vi "LocateDevices.vi"() -> ()   [LabVIEW 2017]
uses:
  D:/upwork/Laser Measurement Tool/Topas4PublicAPI/NET_SDK/Topas4Lib.dll
  Topas4PublicAPI/NET_SDK/Topas4Lib.dll
panel:
  out "Found devices info:":T1(array[cluster])
  out "OPA devices found:":i32
  # "Find OPA device test"
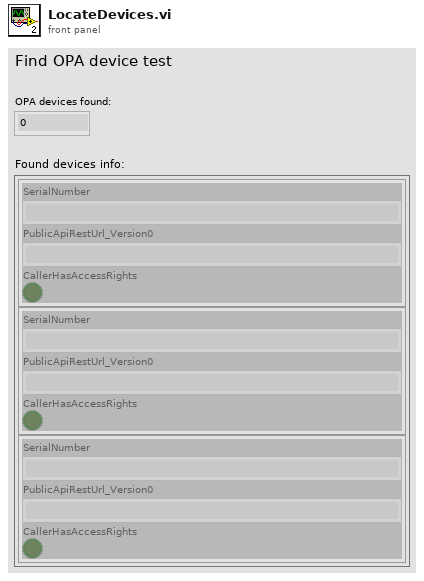
[diagram p1: front panel]
types:
  T1 = cluster{"SerialNumber":string, "PublicApiRestUrl_Version0":string, "CallerHasAccessRights":bool}[]
  T2 = cluster{"SerialNumber":string, "PublicApiRestUrl_Version0":string, "CallerHasAccessRights":bool}
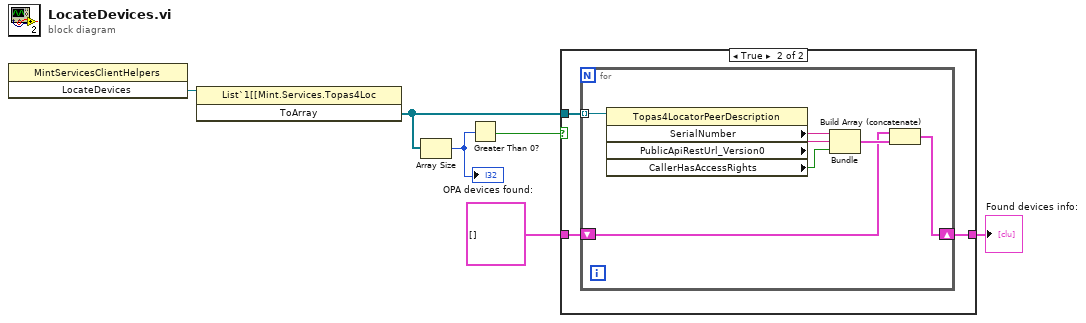
[diagram p0: block diagram]
diagram:
  n1 = invoke class="MintServicesClientHelpers" method="LocateDevices"() -> ("LocateDevices"=w6:refnum<k24>)  [unwired: 3 in, 2 out]
  n2 = invoke class="List`1[[Mint.Services.Topas4Loc" method="ToArray"(reference=w6) -> ("ToArray"=w5:refnum<k24>[])  [unwired: 2 in, 2 out]
  n3 = Array Size(array=w5) -> (size(s)=w4:i32)
  "OPA devices found:" <- w4
  n4 = Greater Than 0?(x=w4) -> (x > 0?=w3:bool)
  n5 = case shown="True" w3 {
    tunnel: w5 -> [_ w10]
    tunnel: T1 [] ("appended array") -> [w7 w9]
    tunnel: [w7 w8] -> w1
    frame False {
    }
    frame True {
      n6 = for {
        tunnel: w10 -> [w17] mode=indexing
        shift-right: [w11] -> w8
        shift-left: w9 -> [w12]
        n7 = property class="Topas4LocatorPeerDescription"(reference=w17) -> ("SerialNumber"=w16:string, "PublicApiRestUrl_Version0"=w15:string, "CallerHasAccessRights"=w14:bool)  [unwired: 1 in, 2 out]
        n8 = Bundle("SerialNumber"=w16, "PublicApiRestUrl_Version0"=w15, "CallerHasAccessRights"=w14) -> (w13:T2)  [unwired: 1 in]
        n9 = Build Array (concatenate)(w12, w13) -> (w11:T1)
      }
    }
  }
  "Found devices info:" <- w1
